vi "Actor Core.vi"(8 "error in":errorcluster, 11 "State in":refnum<class "Receiver Command.lvclass">) -> (0 "error out":errorcluster, 3 "Actor out":refnum<class "Actor.lvclass">)   [LabVIEW 2013]
doc: "(<B>Filename</B>: Actor Framework.lvlib:Actor.lvclass:Actor Core.vi)\n\nThis override invokes Entry.vi on the initial state, prior to calling the parent Actor Core. Adding this behavior to Actor Core (instead of an override of Pre Launch Init.vi) allows the initial state to launch a nested actor as part of its entry behavior.\n\nReceives messages to the actor, reacts to them, and initiates any error handling that may shut the actor down.\n\nDescendant classes may override this VI to append parallel tasks for the actor to complete while it handles messages. Overrides use the Call Parent Method node."
uses:
  <vilib>/ActorFramework/Actor/Actor.lvclass
  Receiver Command.lvclass
  Command/CommandStates.ctl
  Command/Command State Actor.lvclass
  Command/State Status.ctl
  Command Actor/Command States/Command States.lvclass
  Command/Command Status.ctl
  Command Actor/Command Actor.lvclass
panel:
  in  "Command Status":T1
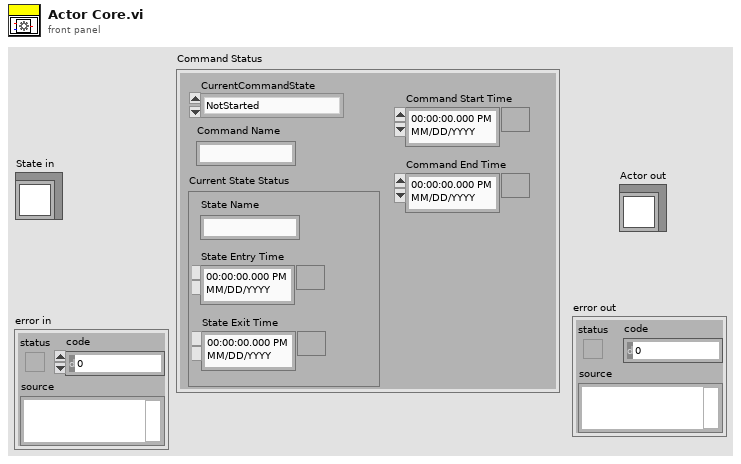
[diagram p1: front panel]
types:
  T1 = typedef "Command Actor.lvlib/Command Actor.lvclass/Command Status.ctl" = cluster{"CurrentCommandState":T2, "Command Name":string, "Current State Status":T3, "Command Start Time":timestamp, "Command End Time":timestamp}
  T2 = typedef "Command State Actor.lvlib/Command State Actor.lvclass/CommandStates.ctl" = enum16{"NotStarted", "Executing", "Stopped", "Completed"}
  T3 = typedef "Command Actor.lvlib/Command States.lvclass/State Status.ctl" = cluster{"State Name":string, "State Entry Time":timestamp, "State Exit Time":timestamp}
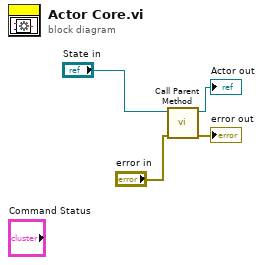
[diagram p0: block diagram]
diagram:
  n1 = call-parent "Call Parent Method"("error in"="error in", "State in"="State in") -> ("error out"=→"error out":errorcluster, "Actor out"=→"Actor out":refnum<class "Actor.lvclass">)  [unwired: 8 in]
